vi "Avantes - AVS_PollScan.vi"(8 "error in (no error)":errorcluster, 11 "AVS Settings In":T1) -> (0 "error out":errorcluster, 2 "Output Ready":i32, 3 "AVS Settings Out":T1)   [LabVIEW 2013, in "Avantes Spectrometer Functions.lvlib"]
uses:
  Avantes Spectrometer Functions.lvlib
  AVS settings.ctl
  IRRAD-DLL/AVSirrad.lvlib
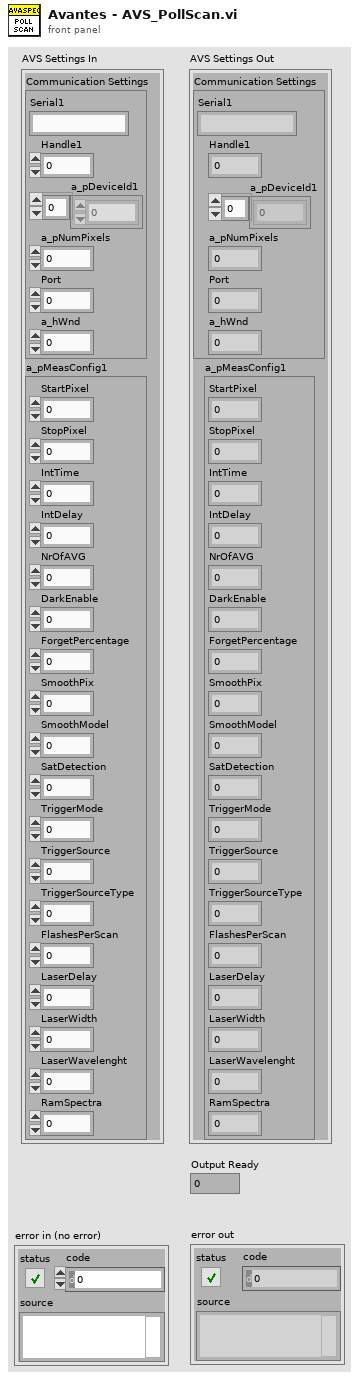
[diagram p1: front panel]
types:
  T1 = typedef "AVSirrad.lvlib/AVS settings.ctl" = cluster{"Communication Settings":cluster{"Serial1":string, "Handle1":i32, "a_pDeviceId1":u8[], "a_pNumPixels":u16, "Port":i32, "a_hWnd":i32}, "a_pMeasConfig1":cluster{"StartPixel":u16, "StopPixel":u16, "IntTime":sgl, "IntDelay":u32, "NrOfAVG":u32, "DarkEnable":u8, "ForgetPercentage":u8, "SmoothPix":u16, "SmoothModel":u8, "SatDetection":u8, "TriggerMode":u8, "TriggerSource":u8, "TriggerSourceType":u8, "FlashesPerScan":u16, "LaserDelay":u32, "LaserWidth":u32, "LaserWavelenght":sgl, "RamSpectra":u16}}
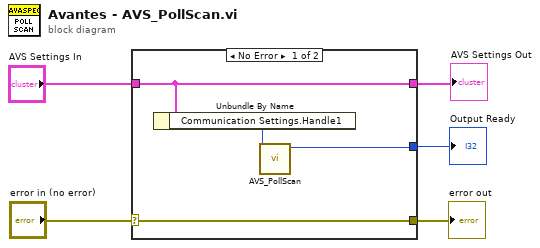
[diagram p0: block diagram]
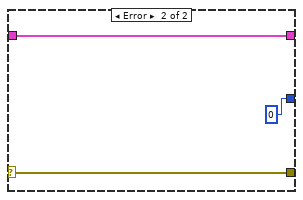
[diagram p2: hidden frame]
diagram:
  n1 = case shown="No Error" "error in (no error)" {
    selector: "error in (no error)" -> [w7 w12]
    tunnel: [w9 w11] -> w1
    tunnel: "AVS Settings In" -> [w9 w11]
    tunnel: [w7 w12] -> w4
    tunnel: [w6 0 ("Output Value")] -> w3
    frame No Error {
      n2 = Unbundle By Name(w9) -> ("Communication Settings.Handle1"=w8:i32)
      n3 = call "AVS_PollScan.vi"("a_hDevice"=w8) -> ("Output Value"=w6:i32)  [unwired: 8 in]
    }
    frame Error {
    }
  }
  "error out" <- w4
  "Output Ready" <- w3
  "AVS Settings Out" <- w1
